vi "Main Page Init SEA FPGA.vi"(8 "error in (no error)":errorcluster, 11 "Item Ref in":T1 format="%.0x") -> (0 "error out":errorcluster, 1 "Current Checksum":string, 2 "Original Checksum":string, 3 "Item Ref out":T1 format="%.0x", 5 "FPGA Name":string)   [LabVIEW 2012, in "AIT 429 System Explorer.lvlib"]
uses:
  AIT 429 System Explorer.lvlib
  <vilib>/NI Veristand/Custom Device API/Custom Device Item Ref.ctl
  Shared/Controls and Global/Global.vi
  <vilib>/NI Veristand/Custom Device API/Get Item Property (String).vi
  <vilib>/NI Veristand/Custom Device API/Get Item Property (Boolean).vi
  <vilib>/NI Veristand/Custom Device API/Get Item Property (Dependent File).vi
  <vilib>/rvi/Utilities/XML/nirviXML_GetValue.vi
  <vilib>/rvi/Utilities/XML/nirviXML_GetValue_String.vi
  <vilib>/NI Veristand/Custom Device API/Get Item Property (Dependent Node Pointer).vi
  <vilib>/NI Veristand/Custom Device API/Custom Device API.lvlib
  <userlib>/_FPGA Interface Advanced Tools/FPGA Bitfile Utility/FPGA Bitfile Utility.lvlib
  Shared/ARINC 429 Shared.lvlib
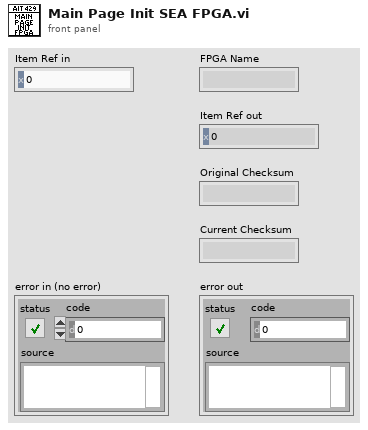
[diagram p1: front panel]
types:
  T1 = typedef "Custom Device API.lvlib/Custom Device Item Ref.ctl" = u64
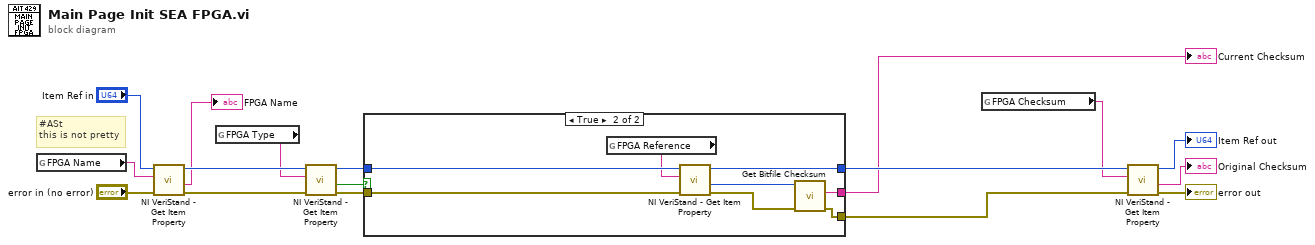
[diagram p0: block diagram]
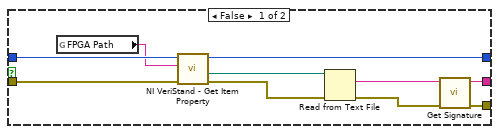
[diagram p2: hidden frame]
diagram:
  # "#ASt\nthis is not pretty"
  n1 = global read "Global.vi" "FPGA Name"() -> (w3:string)
  n2 = call-poly <vilib>:"NI VeriStand - Get Item Property.vi"("error in (no error)"="error in (no error)", "Property Name"=w3, "Item Ref in"="Item Ref in") -> ("error out"=w8:errorcluster, "Value"=→"FPGA Name":string, "Item Ref out"=w9:T1)  [unwired: 5 in, 1 out]
  n3 = global read "Global.vi" "FPGA Type"() -> (w2:string)
  n4 = call-poly <vilib>:"NI VeriStand - Get Item Property.vi"("error in (no error)"=w8, "Property Name"=w2, "Item Ref in"=w9) -> ("error out"=w5:errorcluster, "Value"=w7:bool, "Item Ref out"=w6:T1)  [unwired: 5 in, 1 out]
  n5 = case shown="True" w7 {
    tunnel: [w19 w35] -> w13
    tunnel: [w25 w29] -> w12
    tunnel: [w24 w30] -> w11
    tunnel: w6 -> [w27 w34]
    tunnel: w5 -> [w26 w33]
    frame False {
      n6 = global read "Global.vi" "FPGA Path"() -> (w18:string)
      n7 = call-poly <vilib>:"NI VeriStand - Get Item Property.vi"("error in (no error)"=w26, "Property Name"=w18, "Item Ref in"=w27) -> ("error out"=w23:errorcluster, "Path"=w21:path, "Item Ref out"=w19:T1)  [unwired: 4 in, 2 out]
      n8 = Read from Text File(file (use dialog)=w21, error in=w23) -> (text=w22:string, error out=w20:errorcluster)  [unwired: 2 in, 2 out]
      n9 = call <userlib>:"Get Signature.vi"("error in (no error)"=w20, "bitfile xml in"=w22) -> ("error out"=w25:errorcluster, "Bitfile Signature"=w24:string)  [unwired: 7 in, 1 out]
    }
    frame True {
      n10 = global read "Global.vi" "FPGA Reference"() -> (w28:string)
      n11 = call-poly <vilib>:"NI VeriStand - Get Item Property.vi"("error in (no error)"=w33, "Property Name"=w28, "Item Ref in"=w34) -> ("error out"=w31:errorcluster, "Dependent Node Ref"=w32:T1, "Item Ref out"=w35:T1)  [unwired: 5 in, 1 out]
      n12 = call "Get Bitfile Checksum.vi"("error in (no error)"=w31, "ID in"=w32) -> ("error out"=w29:errorcluster, "MD5"=w30:string)  [unwired: 6 in, 2 out]
    }
  }
  "Current Checksum" <- w11
  n13 = global read "Global.vi" "FPGA Checksum"() -> (w1:string)
  n14 = call-poly <vilib>:"NI VeriStand - Get Item Property.vi"("error in (no error)"=w12, "Property Name"=w1, "Item Ref in"=w13) -> ("error out"=→"error out":errorcluster, "Value"=→"Original Checksum":string, "Item Ref out"=→"Item Ref out":T1)  [unwired: 5 in, 1 out]
